vi "initialise.vi"(8 "error in (no error)":errorcluster, 11 "GenericTrajectory in":refnum<class "TrajectoryDL091126GenericVoxel.lvclass">) -> (0 "error out":errorcluster, 3 "GenericTrajectory out":refnum<class "TrajectoryDL091126GenericVoxel.lvclass">)   [LabVIEW 2010, in "TrajectoryDL091126GenericVoxel.lvclass"]
uses:
  TrajectoryDL091126GenericVoxel.lvclass
  GenericTrajectory/GenericTrajectory/GenericTrajectory.lvclass
  TrajectoryDL091126GenericVoxel.lvclass/TrajectoryDL091126GenericVoxel.ctl
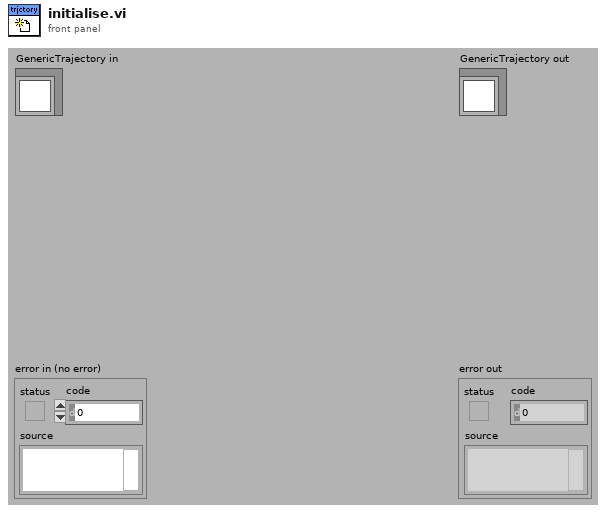
[diagram p1: front panel]
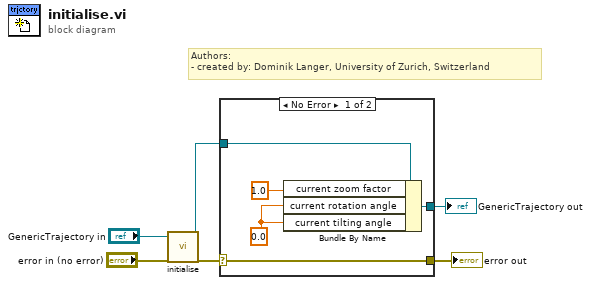
[diagram p0: block diagram]
diagram:
  # "Authors: \n- created by: Dominik Langer, University of Zurich, Switzerland"
  n1 = call-parent "initialise.vi"("error in (no error)"="error in (no error)", "GenericPlugin in"="GenericTrajectory in") -> ("error out"=w3:errorcluster, "GenericPlugin out"=w1:refnum<class "TrajectoryDL091126GenericVoxel.lvclass">)  [unwired: 8 out]
  n2 = case shown="No Error" w3 {
    selector: w3 -> [w7 w13]
    tunnel: [w7 w13] -> w6
    tunnel: [w8 w12] -> w5
    tunnel: w1 -> [w11 w12]
    frame No Error {
      w9 = dbl[unit] 0.0 ("current rotation angle")
      n3 = Bundle By Name(cluster=w11, "current zoom factor"=1.0, "current rotation angle"=w9, "current tilting angle"=w9) -> (w8:refnum<class "TrajectoryDL091126GenericVoxel.lvclass">)
    }
    frame Error {
    }
  }
  "error out" <- w6
  "GenericTrajectory out" <- w5
